vi "main_test2.vi"() -> ()   [LabVIEW 2018]
uses:
  <vilib>/addons/database/Connection.llb/DB Tools Open Connec (Path).vi
  <vilib>/addons/database/NI_Database_API.lvlib
panel:
  in  "head":string
  out "时间":timestamp format="%<%H:%M:%S\n%Y/%m/%d>T"
  out "数据采集":bool=TRUE
  out "flaginit":bool=TRUE
  out "温度报警":string[][](table)
  out "疫苗信息":string[][](table)
  out "uid":i16
  out "途径地点":i32
  out "运输路径":cluster{"city":string, "布尔":T1}[](array[cluster])
  out "error out":errorcluster
  out "负责人信息":T2
  in  "CYJ":bool
  out "定位":bool
  out "温度":sgl(graph)
  out "纬度":string
  out "经度":string
  in  "地图比例":i8(slide)=10 scale=6.0..18.0
  in  "地图":refnum<k7>(container) caption="网页浏览器"
  in  "Setvi":bool
  in  "停止":bool
  # "疫苗冷链储运监控系统\nVACCINE COLD-CHAIN TRANSPORTATION MONITORING SYSTEM"
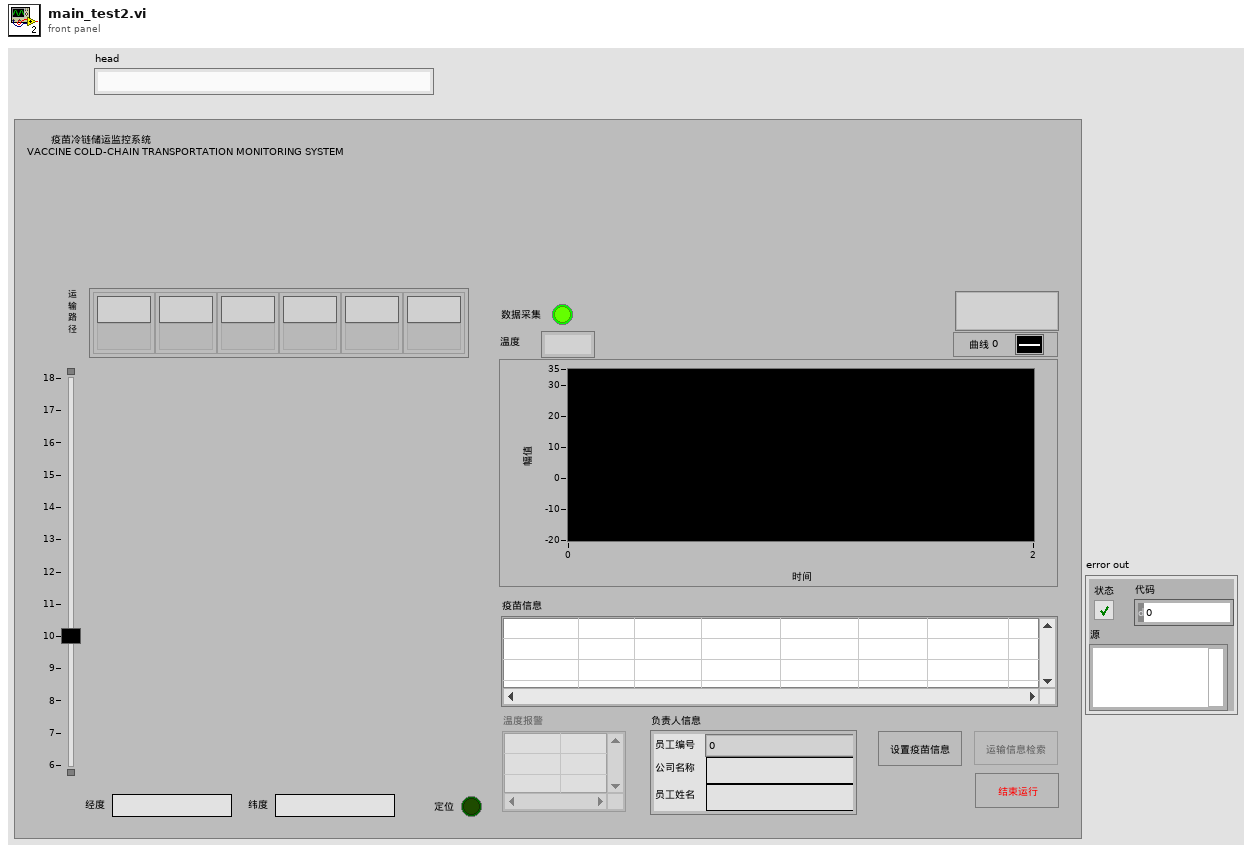
[diagram p1: front panel]
types:
  T1 = typedef "car.ctl" = bool
  T2 = typedef "人员信息.ctl" = cluster{"员工编号":i32, "公司名称":string, "员工姓名":string}
  T3 = typedef "储运信息.ctl" = cluster{"纬度":sgl, "经度":sgl, "温度":sgl, "负责人":i32, "区域":string, "记录时间":timestamp}
  T4 = enum8{"Enabled", "Disabled", "Disabled and Grayed Out"}
  T5 = typedef "NI_Database_API.lvlib/Conn ObjectReference.ctl" = refnum<k1>
  T6 = typedef "疫苗信息.ctl" = cluster{"疫苗名":string, "疫苗编号":i32, "疫苗类型":string, "生产厂家":string, "生产日期":timestamp, "生产地":string, "生产负责人":string, "是否合格":string, "疫苗功能":string}
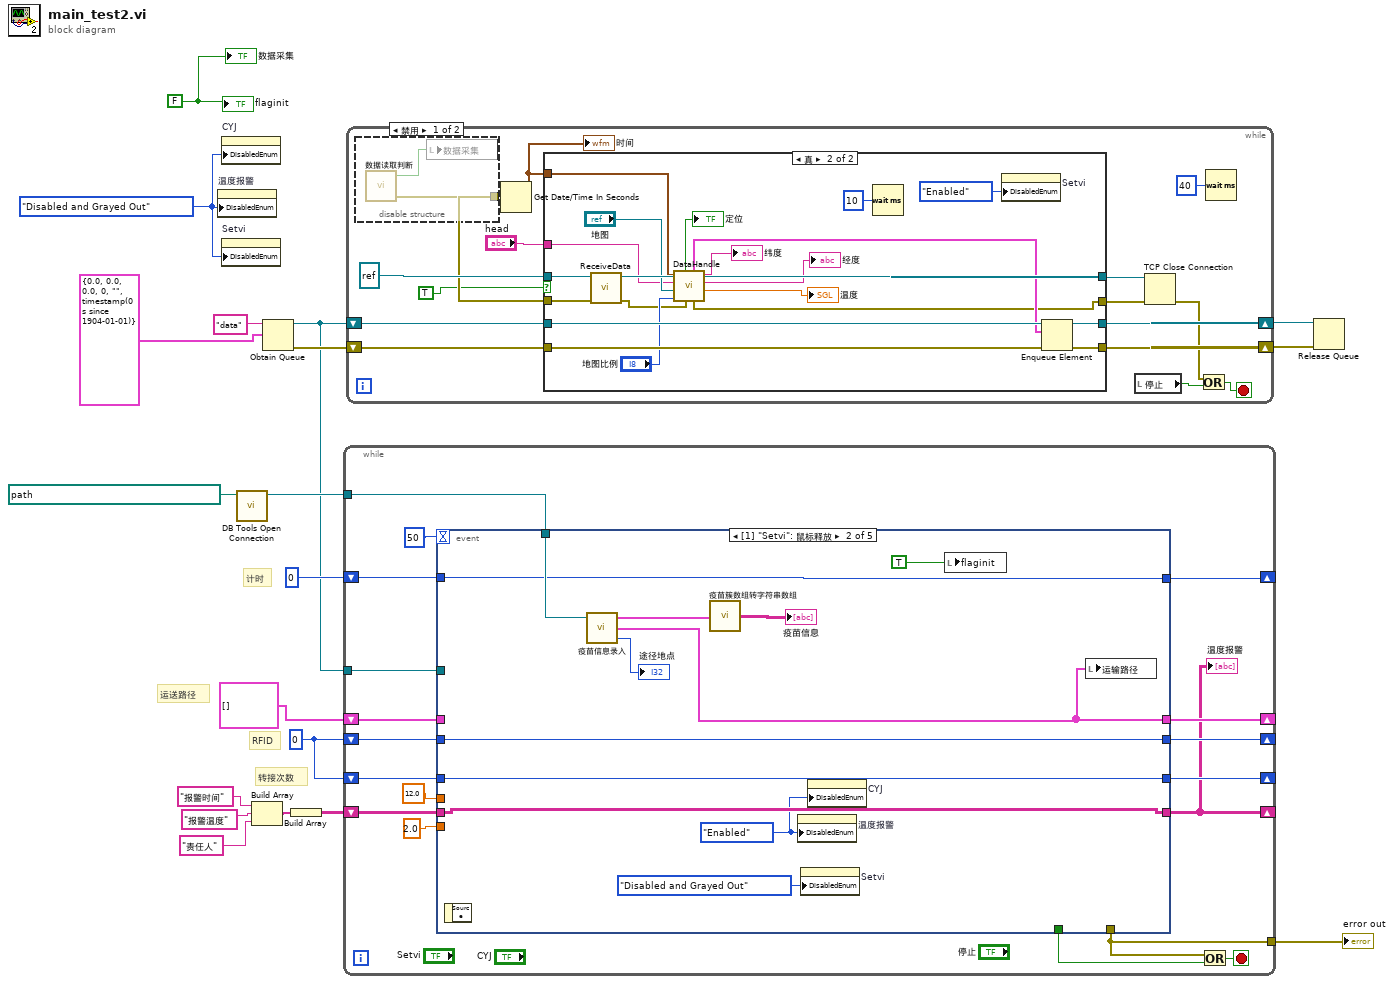
[diagram p0: block diagram]
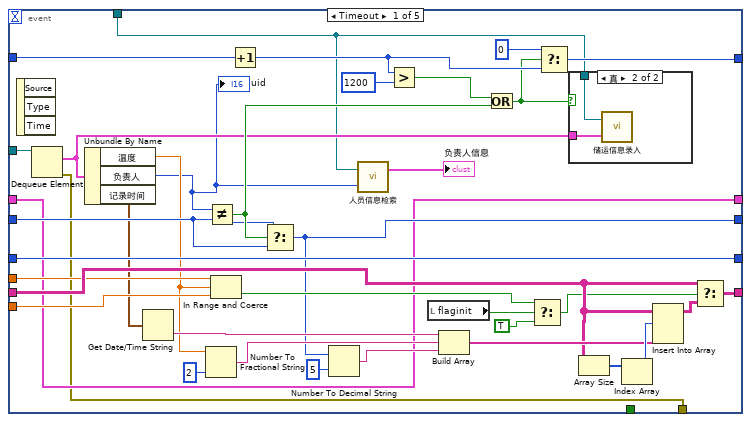
[diagram p2: hidden frame]
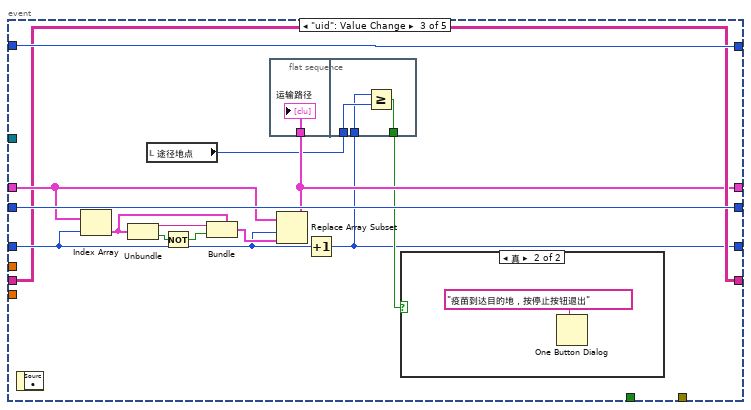
[diagram p4: hidden frame]
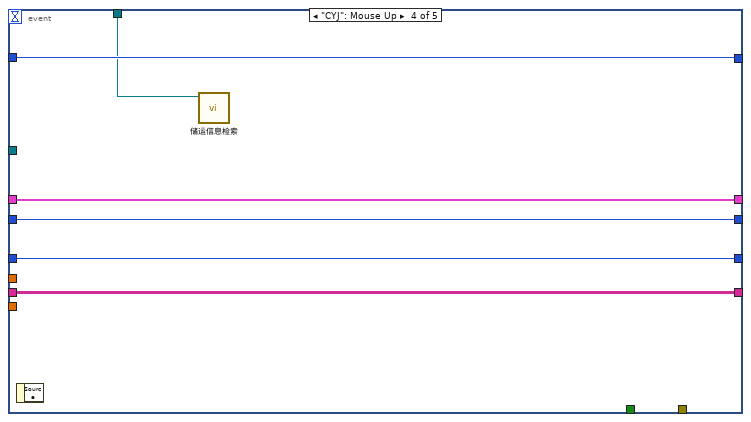
[diagram p6: hidden frame]
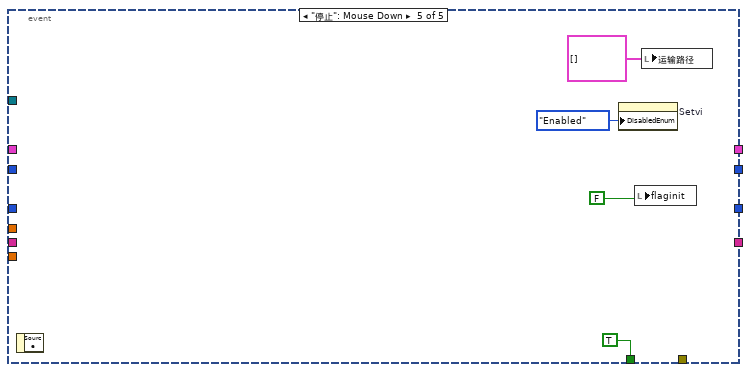
[diagram p7: hidden frame]
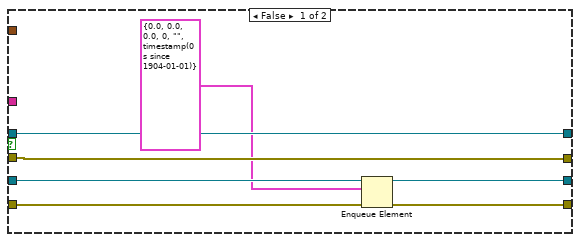
[diagram p9: hidden frame]
diagram:
  w2 = T4."Disabled and Grayed Out" ("禁用")
  w5 = FALSE
  w11 = 0
  # "运送路径"
  # "转接次数"
  # "RFID"
  # "计时"
  n1 = property on="温度报警" class="Tbl (严格)"("DisabledEnum"=w2) -> ()  [unwired: 2 in, 2 out]
  n2 = property on="CYJ" class="Bool (严格)"("DisabledEnum"=w2) -> ()  [unwired: 2 in, 2 out]
  n3 = property on="Setvi" class="Bool (严格)"("DisabledEnum"=w2) -> ()  [unwired: 2 in, 2 out]
  n4 = call-poly <vilib>:"DB Tools Open Connection.vi"("connection information"=path "D:/2019毕业设计/Code/GPData.udl" ("路径")) -> ("connection reference"=w14:T5)  [unwired: 7 in, 1 out]
  n5 = Build Array("报警时间", "报警温度", "责任人") -> (w8:string[])
  n6 = Obtain Queue(name (unnamed)="data" ("名称（未命名）"), element data type=T3 {"纬度"=0.0, "经度"=0.0, "温度"=0.0, "负责人"=0, "区域"="", "记录时间"=timestamp(0 s since 1904-01-01)} ("储运信息簇")) -> (queue out=w4:refnum<queue>, error out=w18:errorcluster)  [unwired: 3 in, 1 out]
  n7 = Build Array(w8) -> (w7:string[][])
  n8 = while {
    tunnel: w14 -> [w37]
    shift-right: [w35] -> _
    shift-left: 0 -> [w34]
    shift-right: [w33] -> _
    shift-left: w11 -> [w32]
    tunnel: [w29] -> w12
    shift-right: [w28] -> _
    shift-left: w11 -> [w27]
    shift-right: [w25] -> _
    shift-left: cluster{string, bool}[] [] -> [w26]
    shift-right: [w21] -> _
    shift-left: w7 -> [w22]
    tunnel: w4 -> [w20]
    stop <- w30 stop-if-true
    n9 = event shown="[1] \"Setvi\": 鼠标释放" {
      selector: _ -> [_ _ _ _ _]
      dyn-events: _ -> [_ _ _ _ _]
      timeout: 50 -> [_ _ _ _ _]
      tunnel: w37 -> [w41 w88 _ w108 _]
      tunnel: [_ _ _ _ TRUE] -> w31
      tunnel: [w71 w87 w102 w113 _] -> w35
      tunnel: w34 -> [w74 w87 w102 w113 _]
      tunnel: [w45 w86 w101 w111 _] -> w33
      tunnel: w32 -> [w68 w86 w101 w111 _]
      tunnel: [w38 _ _ _ _] -> w29
      tunnel: [w69 w84 w89 w110 _] -> w28
      tunnel: w27 -> [w69 w84 w94 w110 _]
      tunnel: [w42 w83 w92 w112 _] -> w25
      tunnel: w26 -> [w42 _ w96 w112 _]
      tunnel: sgl 12.0 ("上限") -> [w51 _ _ _ _]
      tunnel: sgl 2.0 ("下限") -> [w50 _ _ _ _]
      tunnel: w22 -> [w57 w80 w93 w109 _]
      tunnel: [w64 w80 w93 w109 _] -> w21
      tunnel: w20 -> [w49 _ _ _ _]
      event Timeout {
        n10 = event-data() -> ()  [unwired: 1 in, 3 out]
        n11 = Dequeue Element(queue=w49) -> (element=w48:T3, error out=w38:errorcluster)  [unwired: 2 in, 2 out]
        n12 = Unbundle By Name(w48) -> ("温度"=w47:sgl, "负责人"=w40:i32, "记录时间"=w46:timestamp)
        "uid" <- w40
        n13 = Get Date/Time String(seconds (now)=w46) -> (time string=w52:string)  [unwired: 2 in, 1 out]
        n14 = Number To Fractional String(number=w47, precision (6)=i16 2 ("精度(6)")) -> (F-format string=w60:string)  [unwired: 2 in]
        n15 = Not Equal?(x=w40, y=w68) -> (x != y?=w66:bool)
        n16 = In Range and Coerce(upper limit=w51, x=w47, lower limit=w50) -> (In Range?=w55:bool)  [unwired: 1 out]
        n17 = Increment(x=w74) -> (x+1=w72:i32)
        n18 = Select(t=w40, s=w66, f=w68) -> (s? t:f=w45:i32)
        n19 = Number To Decimal String(number=w45, width (-)=i16 5 ("宽度(-)")) -> (decimal integer string=w44:string)
        n20 = call "人员信息检索.vi"("工作人员编号"=w40, "connection reference"=w41) -> ("负责人数据"=→"负责人信息":T2)  [unwired: 1 out]
        n21 = Greater?(x=w72, y=1200) -> (0:w67:bool)
        n22 = local read "flaginit"() -> (w56:bool)
        n23 = Build Array(w52, w60, w44) -> (w59:string[])
        n24 = Or(x=w67, y=w66) -> (x .or. y?=w65:bool)
        n25 = Select(t=w55, s=w56, f=TRUE) -> (s? t:f=w53:bool)
        n26 = Select(t=0, s=w65, f=w72) -> (s? t:f=w71:i32)
        n27 = case shown="真" w65 {
          tunnel: w41 -> [_ w76]
          tunnel: w48 -> [_ w75]
          frame False {
          }
          frame True {
            n28 = call "储运信息录入.vi"("簇"=w75, "connection reference"=w76) -> ()  [unwired: 1 out]
          }
        }
        n29 = Array Size(array=w57) -> (size(s)=w63:i32[])
        n30 = Index Array(array=w63) -> (element=w62:i32)  [unwired: 1 in]
        n31 = Insert Into Array(array=w57, index (row)=w62, new element=w59) -> (w58:string[][])  [unwired: 1 in]
        n32 = Select(t=w57, s=w53, f=w58) -> (s? t:f=w64:string[][])
      }
      event "Setvi": Mouse Up {
        w77 = T4."Enabled" ("禁用")
        n33 = event-data() -> ()  [unwired: 1 in, 1 out]
        n34 = call "疫苗信息录入.vi"("connection"=w88) -> ("途径地点"=→"途径地点":i32, "运输路线"=w83:cluster{"城市":string, bool}[], "疫苗信息"=w82:T6[])  [unwired: 2 in]
        n35 = call "疫苗簇数组转字符串数组.vi"("疫苗信息"=w82) -> ("疫苗信息"=→"疫苗信息":string[][])
        n36 = property on="温度报警" class="Tbl (严格)"("DisabledEnum"=w77) -> ()  [unwired: 2 in, 2 out]
        n37 = property on="Setvi" class="Bool (严格)"("DisabledEnum"=T4."Disabled and Grayed Out" ("禁用")) -> ()  [unwired: 2 in, 2 out]
        n38 = property on="CYJ" class="Bool (严格)"("DisabledEnum"=w77) -> ()  [unwired: 2 in, 2 out]
        n39 = local write "flaginit"(TRUE) -> ()
        n40 = local write "运输路径"(w83) -> ()
      }
      event "uid": Value Change {
        n41 = event-data() -> ()  [unwired: 1 in, 1 out]
        n42 = Index Array(array=w96, index=w94) -> (element=w97:cluster{string, bool})
        n43 = Unbundle(w97) -> (w98:string, w100:bool)
        n44 = local read "途径地点"() -> (w91:i32)
        n45 = Not(x=w100) -> (.not. x?=w99:bool)
        n46 = Bundle(cluster=w97, w98, w99) -> (w95:cluster{string, bool})
        n47 = flat-sequence {
          tunnel: w92 -> [w103]
          tunnel: w91 -> [w106]
          tunnel: [w105] -> w90
          tunnel: w89 -> [w104]
          frame #0 {
            "运输路径" <- w103
          }
          frame #1 {
            n48 = Greater Or Equal?(x=w104, y=w106) -> (x >= y?=w105:bool)
          }
        }
        n49 = Replace Array Subset(array=w96, new element=w95, index=w94) -> (w92:cluster{string, bool}[])
        n50 = Increment(x=w94) -> (x+1=w89:i32)
        n51 = case shown="真" w90 {
          frame False {
          }
          frame True {
            n52 = One Button Dialog(message="疫苗到达目的地，按停止按钮退出" ("消息")) -> ()  [unwired: 1 in, 1 out]
          }
        }
      }
      event "CYJ": Mouse Up {
        n53 = event-data() -> ()  [unwired: 1 in, 1 out]
        n54 = call "储运信息检索.vi"("connection reference"=w108) -> ()  [unwired: 3 in, 3 out]
      }
      event "停止": Mouse Down {
        n55 = event-data() -> ()  [unwired: 1 in, 1 out]
        n56 = property on="Setvi" class="Bool (严格)"("DisabledEnum"=T4."Enabled" ("禁用")) -> ()  [unwired: 2 in, 2 out]
        n57 = local write "flaginit"(FALSE) -> ()
        n58 = local write "运输路径"(cluster{string, bool}[] []) -> ()
      }
    }
    "温度报警" <- w21
    n59 = Or(x=w29, y=w31) -> (x .or. y?=w30:bool)
  }
  "error out" <- w12
  n60 = while {
    shift-right: [w130] -> w17
    shift-left: w4 -> [w132]
    shift-right: [w129] -> w16
    shift-left: w18 -> [w131]
    stop <- w122 stop-if-true
    n61 = disable-structure shown="禁用" {
      disable-tunnel: [w134 _] -> w126
      frame Disabled {
        n62 = call "数据读取判断.vi"() -> ("error out"=w134:errorcluster, "判断错误"=w133:bool)  [unwired: 1 out]
        n63 = local write "数据采集"(w133) -> ()
      }
      frame Enabled {
      }
    }
    n64 = Get Date/Time In Seconds() -> (seconds since 1Jan1904=w121:timestamp)
    "时间" <- w121
    n65 = case shown="真" TRUE {
      tunnel: w132 -> [w138 w161]
      tunnel: w131 -> [w136 w160]
      tunnel: [w137 w159] -> w129
      tunnel: [w139 w158] -> w130
      tunnel: refnum<k5> refnum ("connection ID") -> [w141 w157]
      tunnel: [w141 w156] -> w127
      tunnel: w126 -> [w140 w155]
      tunnel: [w140 w147] -> w125
      tunnel: w121 -> [_ w153]
      tunnel: "head" -> [_ w142]
      frame False {
        n66 = Enqueue Element(queue=w138, element=T3 {"纬度"=0.0, "经度"=0.0, "温度"=0.0, "负责人"=0, "区域"="", "记录时间"=timestamp(0 s since 1904-01-01)} ("储运信息簇"), error in (no error)=w136) -> (queue out=w139:refnum<queue>, error out=w137:errorcluster)  [unwired: 1 in, 1 out]
      }
      frame True {
        n67 = call "ReceiveData.vi"("错误输入（无错误）"=w155, "连接ID"=w157) -> ("错误输出"=w148:errorcluster, "连接ID输出"=w156:refnum<k5>)  [unwired: 5 in, 3 out]
        n68 = call "DataHandle.vi"("error IO"=w148, "滑动杆"="地图比例", "地图"="地图", "data"=w142, "时间"=w153) -> ("温度"=→"温度":sgl, "经度显示"=→"经度":string, "纬度显示"=→"纬度":string, "错误输出"=w147:errorcluster, "储运信息簇"=w151:T3, "定位"=→"定位":bool)  [unwired: 1 out]
        n69 = Wait (ms)(milliseconds to wait=u32 10 ("等待时间（毫秒）")) -> ()  [unwired: 1 out]
        n70 = property on="Setvi" class="Bool (严格)"("DisabledEnum"=T4."Enabled" ("禁用")) -> ()  [unwired: 2 in, 2 out]
        n71 = Enqueue Element(queue=w161, element=w151, error in (no error)=w160) -> (queue out=w158:refnum<queue>, error out=w159:errorcluster)  [unwired: 1 in, 1 out]
      }
    }
    n72 = local read "停止"() -> (w123:bool)
    n73 = TCP Close Connection(connection ID=w127, error in (no error)=w125) -> (error out=w124:errorcluster)  [unwired: 1 in, 1 out]
    n74 = Or(x=w124, y=w123) -> (x .or. y?=w122:bool)
    n75 = Wait (ms)(milliseconds to wait=u32 40 ("等待时间（毫秒）")) -> ()  [unwired: 1 out]
  }
  n76 = Release Queue(queue=w17, error in (no error)=w16) -> ()  [unwired: 1 in, 3 out]
  "flaginit" <- w5
  "数据采集" <- w5
